vi "SendDataLogTele.vi"(0 "Cluster":cluster{"chat_id":string, "text":string}) -> ()   [LabVIEW 2021]
uses:
  <vilib>/httpClient/POSTBuffer.vi
  <vilib>/httpClient/LabVIEWHTTPClient.lvlib
panel:
  out "error out":errorcluster
  out "body":string
  out "headers":string
  out "JSON string":string
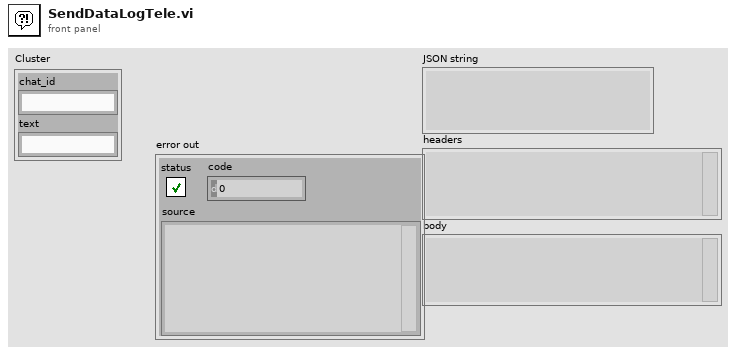
[diagram p1: front panel]
types:
  T1 = typedef "LabVIEWHTTPClient.lvlib/ClientHandle.ctl" = refnum<k1>
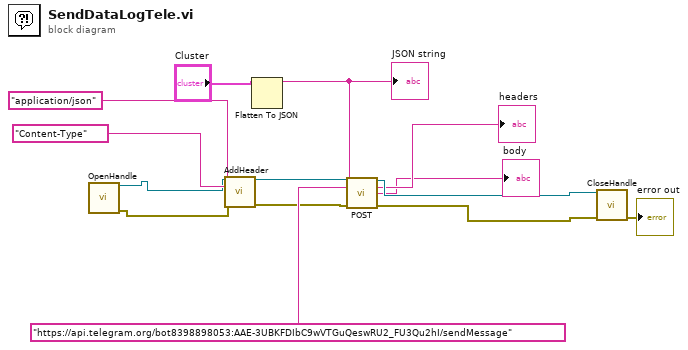
[diagram p0: block diagram]
diagram:
  n1 = call <vilib>:"OpenHandle.vi"() -> ("client handle out"=w2:T1, "error out"=w1:errorcluster)  [unwired: 14 in]
  n2 = call <vilib>:"AddHeader.vi"("client handle"=w2, "header"="Content-Type", "value"="application/json", "error in (no error)"=w1) -> ("client handle out"=w11:T1, "error out"=w5:errorcluster)  [unwired: 10 in]
  n3 = Flatten To JSON(anything="Cluster") -> (JSON string=w4:string)  [unwired: 2 in, 1 out]
  "JSON string" <- w4
  n4 = call-poly <vilib>:"POST.vi"("client handle"=w11, "url"="https://api.telegram.org/bot8398898053:AAE-3UBKFDIbC9wVTGuQeswRU2_FU3Qu2hI/sendMessage", "buffer"=w4, "error in (no error)"=w5) -> ("client handle out"=w13:T1, "headers"=→"headers":string, "body"=→"body":string, "error out"=w12:errorcluster)  [unwired: 8 in]
  n5 = call <vilib>:"CloseHandle.vi"("client handle"=w13, "error in (no error)"=w12) -> ("error out"=→"error out":errorcluster)  [unwired: 13 in]
